vi "Log data.vi"(8 "error in (no error)":errorcluster, 11 "Results":T1) -> (0 "error out":errorcluster, 2 "log file path":path, 3 "log file name":string)   [LabVIEW 2019]
doc: "Logs results from the test. Note that this VI currently logs all data at once at end of test. This means we need to aggregate data from individual tests into an array of clusters (probably via FGV, possible queue) before passing the data to the final step of this VI."
uses:
  controls/Log Data Cluster.ctl
  controls/Communication Types.ctl
  controls/Results.ctl
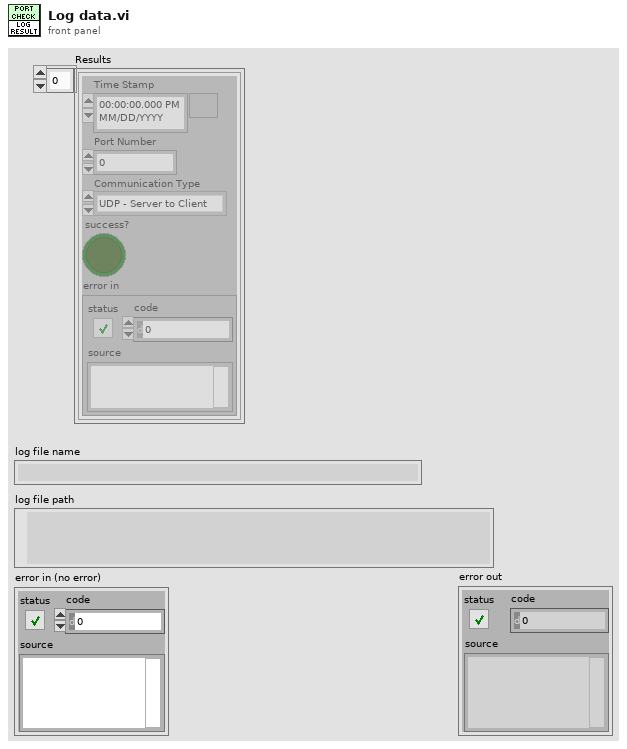
[diagram p1: front panel]
types:
  T1 = typedef "Results.ctl" = T2[]
  T2 = typedef "log data cluster.ctl" = cluster{"Time Stamp":timestamp, "Port Number":u16, "Communication Type":T3, "success?":bool, "error in":errorcluster}
  T3 = typedef "Communication Types.ctl" = enum16{"UDP - Server to Client", "UDP - Client to Server", "TCP - Server to Client", "TCP - Client to Server"}
  T4 = enum16{"open", "replace", "create", "open or create", "replace or create", "replace or create with confirmation"}
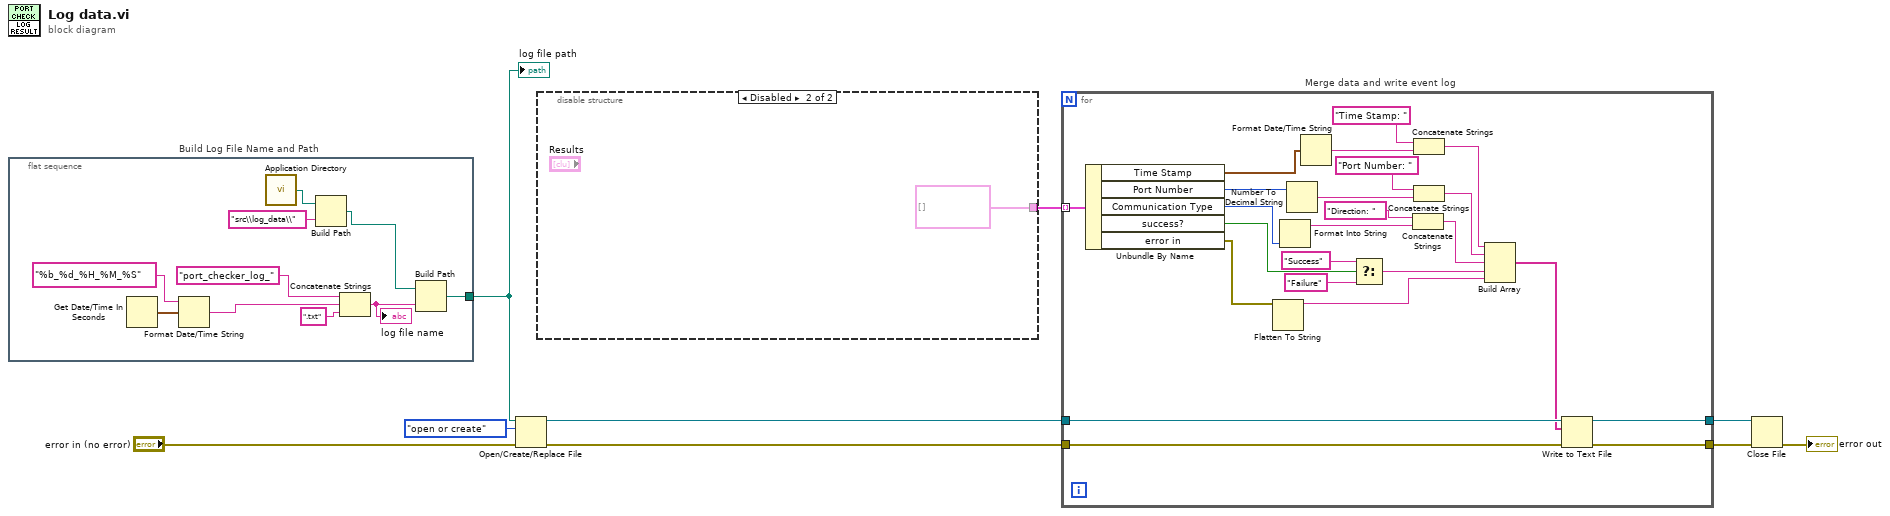
[diagram p0: block diagram]
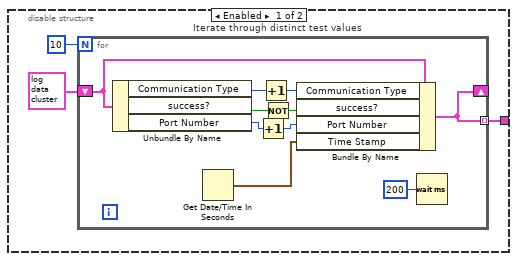
[diagram p2: hidden frame]
diagram:
  n1 = flat-sequence "Build Log File Name and Path" {
    tunnel: [w11] -> w8
    frame #0 {
      n2 = Get Date/Time In Seconds() -> (seconds since 1Jan1904=w19:timestamp)
      n3 = Format Date/Time String(time format string (%c)="%b_%d_%H_%M_%S", seconds (now)=w19) -> (date/time string=w16:string)  [unwired: 1 in]
      n4 = call <vilib>:"Application Directory.vi"() -> ("Application Directory"=w15:path)
      n5 = Build Path(base path=w15, name or relative path="src\\log_data\\") -> (appended path=w13:path)
      n6 = Concatenate Strings("port_checker_log_" ("string"), w16, ".txt" ("string")) -> (w10:string)
      "log file name" <- w10
      n7 = Build Path(base path=w13, name or relative path=w10) -> (appended path=w11:path)
    }
  }
  n8 = Open/Create/Replace File(file path (use dialog)=w8, error in="error in (no error)", operation (0:open)=T4."open or create") -> (refnum out=w7:refnum<file>, error out=w6:errorcluster)  [unwired: 3 in, 1 out]
  n9 = disable-structure shown="Disabled" {
    disable-tunnel: [w20 T1 [] ("Results")] -> w1
    frame Enabled {
      n10 = for "Iterate through distinct test values" {
        N: 10 -> [_]
        shift-right: [w29] -> _
        shift-left: T2 {"Time Stamp"=timestamp(0 s since 1904-01-01), "Port Number"=0, "Communication Type"=enum."UDP - Server to Client", "success?"=FALSE, "error in"={"status"=FALSE, "code"=0, "source"=""}} ("log_data") -> [w31]
        tunnel: [w29] -> w20 mode=indexing
        n11 = Unbundle By Name(w31) -> ("Communication Type"=w32:T3, "success?"=w28:bool, "Port Number"=w24:u16)
        n12 = Get Date/Time In Seconds() -> (seconds since 1Jan1904=w23:timestamp)
        n13 = Increment(x=w24) -> (x+1=w25:u16)
        n14 = Increment(x=w32) -> (x+1=w30:T3)
        n15 = Not(x=w28) -> (.not. x?=w27:bool)
        n16 = Bundle By Name(cluster=w31, "Communication Type"=w30, "success?"=w27, "Port Number"=w25, "Time Stamp"=w23) -> (w29:T2)
        n17 = Wait (ms)(milliseconds to wait=u32 200) -> ()  [unwired: 1 out]
      }
    }
    frame Disabled {
    }
  }
  n18 = for "Merge data and write event log" {
    tunnel: w7 -> [w57]
    tunnel: w6 -> [w56]
    tunnel: w1 -> [w44] mode=indexing
    tunnel: [w48] -> w5
    tunnel: [w47] -> w4
    n19 = Unbundle By Name(w44) -> ("Time Stamp"=w34:timestamp, "Port Number"=w55:u16, "Communication Type"=w54:T3, "success?"=w51:bool, "error in"=w50:errorcluster)
    n20 = Flatten To String(anything=w50) -> (data string=w45:string)  [unwired: 3 in, 2 out]
    n21 = Format Into String(w54) -> (resulting string=w36:string)  [unwired: 3 in, 1 out]
    n22 = Number To Decimal String(number=w55) -> (decimal integer string=w39:string)  [unwired: 1 in]
    n23 = Format Date/Time String(seconds (now)=w34) -> (date/time string=w42:string)  [unwired: 2 in]
    n24 = Select(t="Success", s=w51, f="Failure") -> (s? t:f=w46:string)
    n25 = Concatenate Strings("Direction: " ("string"), w36) -> (w35:string)
    n26 = Concatenate Strings("Time Stamp: " ("string"), w42) -> (w41:string)
    n27 = Concatenate Strings("Port Number: " ("string"), w39) -> (w38:string)
    n28 = Build Array(w41, w38, w35, w46, w45) -> (w49:string[])
    n29 = Write to Text File(file (use dialog)=w57, text=w49, error in=w56) -> (refnum out=w48:refnum<file>, error out=w47:errorcluster)  [unwired: 1 in, 1 out]
  }
  n30 = Close File(refnum=w5, error in=w4) -> (error out=→"error out":errorcluster)  [unwired: 1 out]
  "log file path" <- w8
